vi "Unit Test Mutation (Nested Object).vi"() -> ()   [LabVIEW 2019, in "Sports Unit Tests.lvclass"]
uses:
  Sports Unit Tests.lvclass
  Classes/Bill Murray/Bill Murray.lvclass
  <vilib>/Utility/error.llb/Clear Errors.vi
  <vilib>/addons/_JKI Toolkits/Caraya/classes/Test/Define Test.vi
  <vilib>/addons/_JKI Toolkits/Caraya/classes/Assert/Assert Equal Value_Variant.vi
  <vilib>/addons/_JKI Toolkits/Caraya/classes/Assert/Assert Not Error.vi
  <vilib>/addons/_JKI Toolkits/Caraya/classes/Assert/Assert.lvclass
  Classes/Golf Club.lvclass
  <userlib>/Blue Origin/BlueSerialization/BlueSerializer/BlueSerializer.lvclass
panel:
  out "Table":string[][](table)=[["{\r  \"Class\":[\"Bill Murray.lvclass\",\"Golf Player.lvclass\",\"Sports Player.lvclass\",\"Human.lvclass\",\"BlueSerialization.lvlib:BlueSerializable.lvclass\"],\r  \"Version\":[\"2.0.0.3\",\"2.0.0.3\",\"2.0.0.3\",\"2.0.0.3\",\"2.0.0.0\"],\r  \"BlueSerialization.lvlib:BlueSerializable.lvclass\":{\"LibVersion\":1},\r  \"Human.lvclass\":{\r    \"alive?\":true,\r    \"Age (years)\":40,\r    \"Name\":\"Bill Murray\",\r    \"Height (ft)\":6\r  },\r  \"Sports Player.lvclass\":{\r    \"Professional?\":false,\r    \"Earnings (dollars)\":1000000,\r    \"Sponsor\":\"SNL\"\r  },\r  \"Golf Player.lvclass\":{\r    \"League\":\"Caddyshack League\",\r    \"# holes in one\":-1,\r    \"longest drive (ft)\":-100\r  },\r  \"Bill Murray.lvclass\":{\r    \"Nickname\":\"Carl Spackler\",\r    \"Golf Club\":{\r      \"Class\":[\"Golf Club.lvclass\",\"BlueSerialization.lvlib:BlueSerializable.lvclass\"],\r      \"Version\":[\"2.0.0.3\",\"2.0.0.0\"],\r      \"BlueSerialization.lvlib:BlueSerializable.lvclass\":{\"LibVersion\":1},\r      \"Golf Club.lvclass\":{\"Club Number\":5}\r    }\r  }\r}", "{\r  \"Class\":[\"Bill Murray.lvclass\",\"Golf Player.lvclass\",\"Sports Player.lvclass\",\"Human.lvclass\",\"BlueSerialization.lvlib:BlueSerializable.lvclass\"],\r  \"Version\":[\"2.0.0.3\",\"2.0.0.3\",\"2.0.0.3\",\"2.0.0.3\",\"2.0.0.0\"],\r  \"BlueSerialization.lvlib:BlueSerializable.lvclass\":{\"LibVersion\":1},\r  \"Human.lvclass\":{\r    \"alive?\":true,\r    \"Age (years)\":40,\r    \"Name\":\"Bill Murray\",\r    \"Height (ft)\":6\r  },\r  \"Sports Player.lvclass\":{\r    \"Professional?\":false,\r    \"Earnings (dollars)\":1000000,\r    \"Sponsor\":\"SNL\"\r  },\r  \"Golf Player.lvclass\":{\r    \"League\":\"Caddyshack League\",\r    \"# holes in one\":-1,\r    \"longest drive (ft)\":-100\r  },\r  \"Bill Murray.lvclass\":{\r    \"Nickname\":\"Carl Spackler\",\r    \"Golf Club\":{\r      \"Class\":[\"Golf Club.lvclass\",\"BlueSerialization.lvlib:BlueSerializable.lvclass\"],\r      \"Version\":[\"2.0.0.3\",\"2.0.0.0\"],\r      \"BlueSerialization.lvlib:BlueSerializable.lvclass\":{\"LibVersion\":1},\r      \"Golf Club.lvclass\":{\"Club Number\":5}\r    }\r  }\r}", "Status: FALSE\ncode: 0\n", "BlueJSONTextSerializer.lvlib:BlueJSONTextSerializer.lvclass"], ["Class = [\"Bill Murray.lvclass\", \"Golf Player.lvclass\", \"Sports Player.lvclass\", \"Human.lvclass\", \"BlueSerialization.lvlib:BlueSerializable.lvclass\"]\r\nVersion = [\"2.0.0.3\", \"2.0.0.3\", \"2.0.0.3\", \"2.0.0.3\", \"2.0.0.0\"]\r\n\n[\"BlueSerialization.lvlib:BlueSerializable.lvclass\"]\nLibVersion = 1\r\n\n[\"Human.lvclass\"]\n\"alive?\" = true\r\n\"Age (years)\" = 40\r\nName = \"Bill Murray\"\r\n\"Height (ft)\" = 6.0\r\n\n[\"Sports Player.lvclass\"]\n\"Professional?\" = false\r\n\"Earnings (dollars)\" = 1000000.0\r\nSponsor = \"SNL\"\r\n\n[\"Golf Player.lvclass\"]\nLeague = \"Caddyshack League\"\r\n\"# holes in one\" = -1\r\n\"longest drive (ft)\" = -100.0\r\n\n[\"Bill Murray.lvclass\"]\nNickname = \"Carl Spackler\"\r\n\n[\"Bill Murray.lvclass\".\"Golf Club\"]\nClass = [\"Golf Club.lvclass\", \"BlueSerialization.lvlib:BlueSerializable.lvclass\"]\r\nVersion = [\"2.0.0.3\", \"2.0.0.0\"]\r\n\n[\"Bill Murray.lvclass\".\"Golf Club\".\"BlueSerialization.lvlib:BlueSerializable.lvclass\"]\nLibVersion = 1\r\n\n[\"Bill Murray.lvclass\".\"Golf Club\".\"Golf Club.lvclass\"]\n\"Club Number\" = 5\r\n", "Class = [\"Bill Murray.lvclass\", \"Golf Player.lvclass\", \"Sports Player.lvclass\", \"Human.lvclass\", \"BlueSerialization.lvlib:BlueSerializable.lvclass\"]\r\nVersion = [\"2.0.0.3\", \"2.0.0.3\", \"2.0.0.3\", \"2.0.0.3\", \"2.0.0.0\"]\r\n\n[\"BlueSerialization.lvlib:BlueSerializable.lvclass\"]\nLibVersion = 1\r\n\n[\"Human.lvclass\"]\n\"alive?\" = true\r\n\"Age (years)\" = 40\r\nName = \"Bill Murray\"\r\n\"Height (ft)\" = 6.0\r\n\n[\"Sports Player.lvclass\"]\n\"Professional?\" = false\r\n\"Earnings (dollars)\" = 1000000.0\r\nSponsor = \"SNL\"\r\n\n[\"Golf Player.lvclass\"]\nLeague = \"Caddyshack League\"\r\n\"# holes in one\" = -1\r\n\"longest drive (ft)\" = -100.0\r\n\n[\"Bill Murray.lvclass\"]\nNickname = \"Carl Spackler\"\r\n\n[\"Bill Murray.lvclass\".\"Golf Club\"]\nClass = [\"Golf Club.lvclass\", \"BlueSerialization.lvlib:BlueSerializable.lvclass\"]\r\nVersion = [\"2.0.0.3\", \"2.0.0.0\"]\r\n\n[\"Bill Murray.lvclass\".\"Golf Club\".\"BlueSerialization.lvlib:BlueSerializable.lvclass\"]\nLibVersion = 1\r\n\n[\"Bill Murray.lvclass\".\"Golf Club\".\"Golf Club.lvclass\"]\n\"Club Number\" = 5\r\n", "Status: FALSE\ncode: 0\n", "BlueTOMLSerializer.lvlib:BlueTOMLSerializer.lvclass"]]
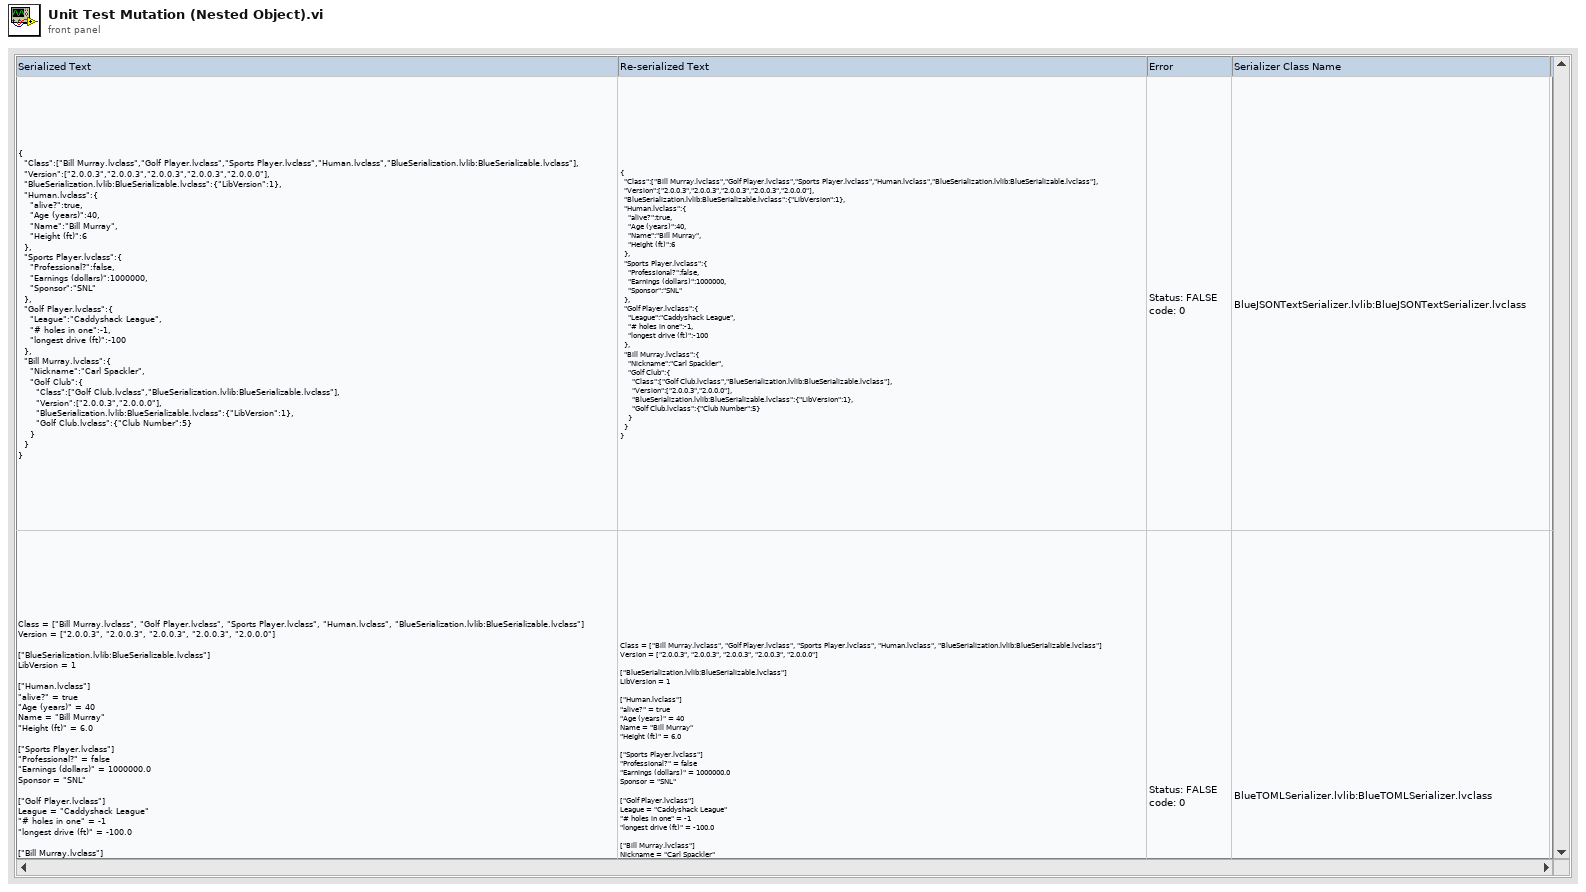
[diagram p1: front panel]
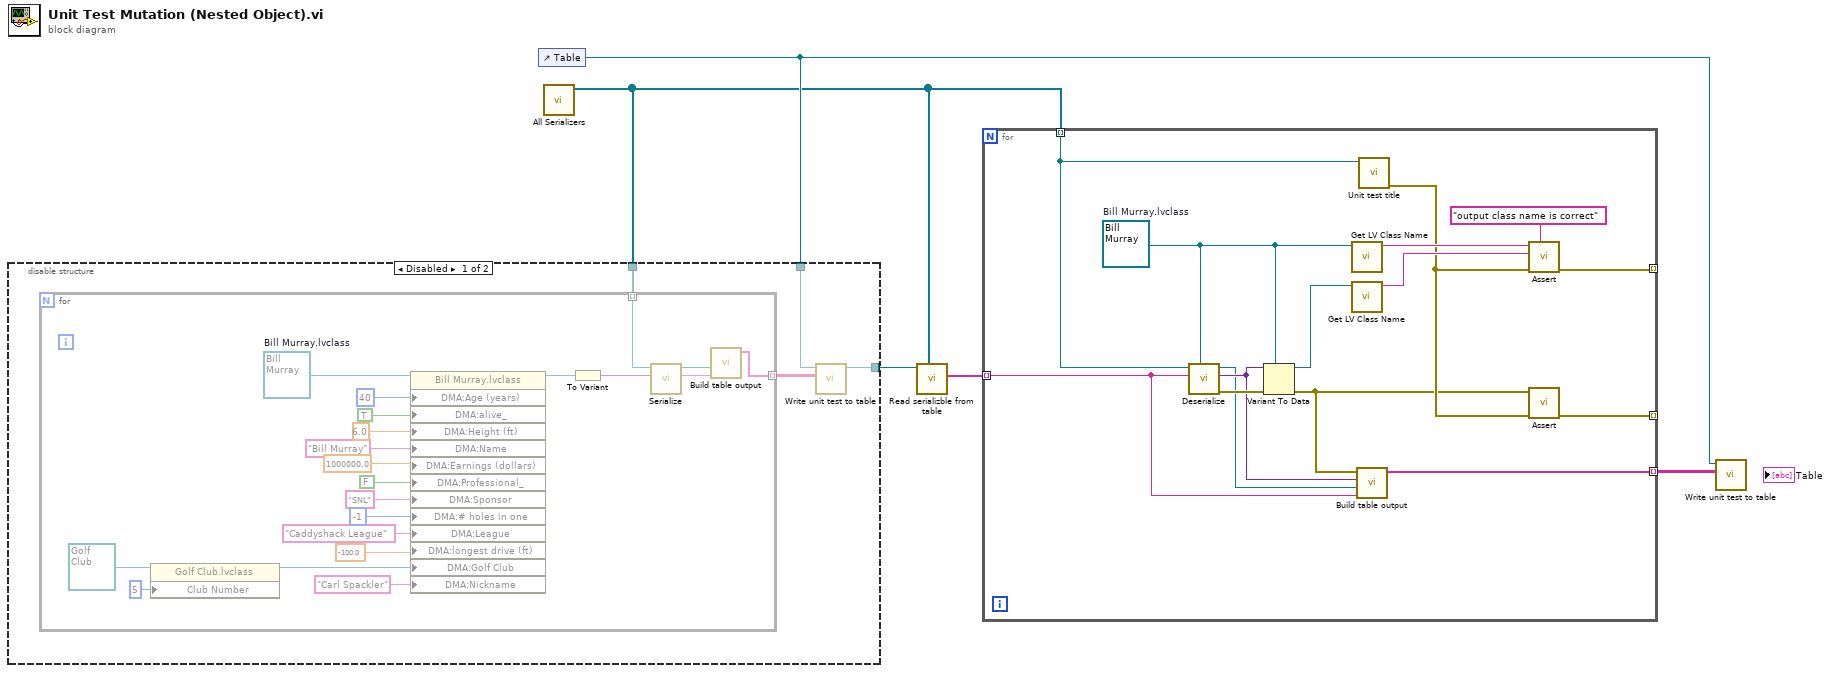
[diagram p0: block diagram]
diagram:
  n1 = control-ref of="Table"() -> (w5:refnum<vi>)
  n2 = call "All Serializers.vi"() -> ("All serializers"=w2:refnum<class "BlueSerializer.lvclass">[])  [unwired: 11 in]
  n3 = disable-structure shown="Disabled" {
    disable-tunnel: w5 -> [w8 w31]
    disable-tunnel: [w7 w31] -> w4
    disable-tunnel: w2 -> [w6 _]
    frame Disabled {
      n4 = for {
        tunnel: w6 -> [w21] mode=indexing
        tunnel: [w18] -> w9 mode=indexing
        w14 = refnum<class "Bill Murray.lvclass"> refnum  # Bill Murray.lvclass
        n5 = property class="Golf Club.lvclass"(reference=refnum<class "Golf Club.lvclass"> refnum ("Golf Club.lvclass"), "Club Number"=5) -> (reference out=w11:refnum<class "Golf Club.lvclass">)  [unwired: 1 in, 1 out]
        n6 = property on="Property Node" class="Bill Murray.lvclass"(reference=w14, "DMA:Age (years)"=u16 40 ("Age (years)"), "DMA:alive_"=TRUE ("alive_"), "DMA:Height (ft)"=6.0 ("Height (ft)"), "DMA:Name"="Bill Murray" ("Name"), "DMA:Earnings (dollars)"=1000000.0 ("Earnings (dollars)"), "DMA:Professional_"=FALSE ("Professional_"), "DMA:Sponsor"="SNL" ("Sponsor"), "DMA:# holes in one"=-1 ("# holes in one"), "DMA:League"="Caddyshack League" ("League"), "DMA:longest drive (ft)"=-100.0 ("longest drive (ft)"), "DMA:Golf Club"=w11, "DMA:Nickname"="Carl Spackler" ("Nickname")) -> (reference out=w30:refnum<class "Bill Murray.lvclass">)  [unwired: 1 in, 1 out]
        n7 = To Variant(anything=w30) -> (Variant=w22:variant)
        n8 = call <userlib>:"Serialize.vi"("Anything"=w22, "BlueSerializer in"=w21) -> ("Serialized Text"=w20:string, "BlueSerializer out"=w19:refnum<class "BlueSerializer.lvclass">)  [unwired: 7 in, 1 out]
        n9 = call "Build table output.vi"("serialized text"=w20, "BlueSerializer in"=w19) -> ("table output"=w18:string[])  [unwired: 9 in]
      }
      n10 = call "Write unit test to table.vi"("Table"=w9, "Table ref in"=w8) -> ("Table ref out"=w7:refnum<vi>)  [unwired: 9 in]
    }
    frame Enabled {
    }
  }
  n11 = call "Read serializble from table.vi"("serializers"=w2, "Table ref in"=w4) -> ("serializable texts"=w3:string[])  [unwired: 7 in, 2 out]
  n12 = for {
    tunnel: w2 -> [w33] mode=indexing
    tunnel: [w41] -> _ mode=indexing
    tunnel: [w40] -> _ mode=indexing
    tunnel: w3 -> [w35] mode=indexing
    tunnel: [w34] -> w1 mode=indexing
    w32 = refnum<class "Bill Murray.lvclass"> refnum  # Bill Murray.lvclass
    n13 = call <userlib>:"Deserialize.vi"("Anything"=w32, "Serialized Text"=w35, "BlueSerializer in"=w33) -> ("error out"=w46:errorcluster, "Variant"=w37:variant, "BlueSerializer out"=w36:refnum<class "BlueSerializer.lvclass">)  [unwired: 6 in]
    n14 = Variant To Data(error in=w46, type=w32, Variant=w37) -> (data=w45:refnum<class "Bill Murray.lvclass">, error out=w38:errorcluster)
    n15 = call <vilib>:"Get LV Class Name.vi"("object"=w32) -> ("class name"=w44:string)  [unwired: 9 in, 1 out]
    n16 = call <vilib>:"Get LV Class Name.vi"("object"=w45) -> ("class name"=w43:string)  [unwired: 9 in, 1 out]
    n17 = call "Build table output.vi"("serialized text"=w35, "BlueSerializer in"=w36, "deserialized variant"=w37, "variant to data error"=w38) -> ("table output"=w34:string[])  [unwired: 7 in]
    n18 = call "Unit test title.vi"("serializer"=w33) -> ("error out"=w39:errorcluster)  [unwired: 9 in, 1 out]
    n19 = call-poly <vilib>:"Assert.vi"("Label"="output class name is correct", "error in (no error)"=w39, "Y"=w43, "X"=w44) -> ("error out"=w40:errorcluster)  [unwired: 7 in]
    n20 = call-poly <vilib>:"Assert.vi"("error in (no error)"=w39, "Not Error?"=w38) -> ("error out"=w41:errorcluster)  [unwired: 9 in]
  }
  n21 = call "Write unit test to table.vi"("Table"=w1, "Table ref in"=w5) -> ()  [unwired: 9 in, 1 out]
